vi "Write configuration.vi"(8 "error in (no error)":errorcluster, 11 "Galvo in":refnum<class "InVivo_ImagingModeSPIM.lvclass">) -> (0 "error out":errorcluster, 3 "Galvo out":refnum<class "InVivo_ImagingModeSPIM.lvclass">)   [LabVIEW 2012, in "InVivo_ImagingModeSPIM.lvclass"]
doc: "Writes the configuration cluster into the configuration file. Configuration file is XML-based. It's name is <component ID>.xml"
uses:
  InVivo_ImagingModeSPIM.lvclass
  <vilib>/Distrio/Murmex/Murmex/Murmex.lvclass
  InVivo_ImagingModeSPIM.lvclass/InVivo_ImagingModeSPIM.ctl
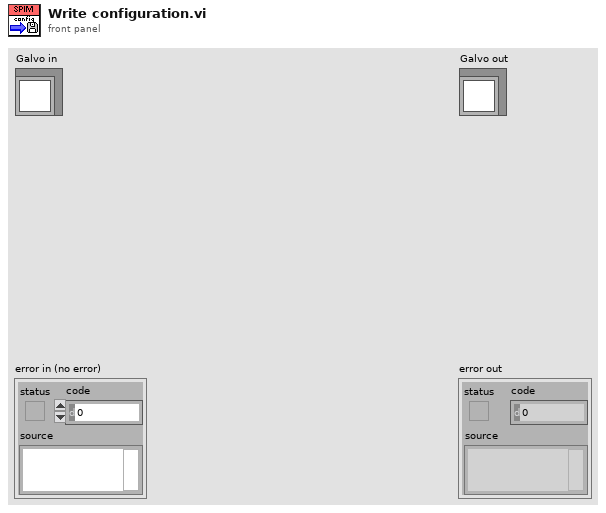
[diagram p1: front panel]
types:
  T1 = typedef "InVivo_ImagingModeSPIM.lvclass/configuration_cluster.ctl" = cluster{"number of channels":u8, "Sampling rate":dbl, "Samples per channel":i32}
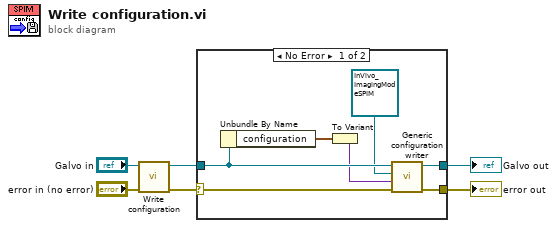
[diagram p0: block diagram]
diagram:
  n1 = call-parent "Write configuration.vi"("error in (no error)"="error in (no error)", "Murmex in"="Galvo in") -> ("error out"=w4:errorcluster, "Murmex out"=w3:refnum<class "InVivo_ImagingModeSPIM.lvclass">)  [unwired: 8 in]
  n2 = case shown="No Error" w4 {
    selector: w4 -> [w13 w14]
    tunnel: w3 -> [w12 w15]
    tunnel: [w8 w15] -> w2
    tunnel: [w7 w14] -> w1
    frame No Error {
      n3 = Unbundle By Name(w12) -> ("configuration"=w11:T1)
      n4 = To Variant(anything=w11) -> (Variant=w10:variant)
      n5 = call <vilib>:"Generic configuration writer.vi"("error in (no error)"=w13, "configuration"=w10, "inheritance level"=refnum<class "InVivo_ImagingModeSPIM.lvclass"> refnum ("Galvo.lvclass"), "MurmexBase in"=w12) -> ("error out"=w7:errorcluster, "MurmexBase out"=w8:refnum<class "InVivo_ImagingModeSPIM.lvclass">)  [unwired: 6 in]
    }
    frame Error {
    }
  }
  "error out" <- w1
  "Galvo out" <- w2
